vi "Virtualni instrument za merenje elektrofizioloskih signala.vi"() -> ()   [LabVIEW 2013]
uses:
  <vilib>/Instr/_visa.llb/VISA Configure Serial Port (Instr).vi
panel:
  out "Graficki prikaz rezultata":dbl(graph)
  in  "?":bool
  in  "Izbor porta":refnum<visa-resource-name>
  out "Broj rezultata":i32
  out "Lokacija sacuvanog fajla na racunaru":path
  in  "?":bool
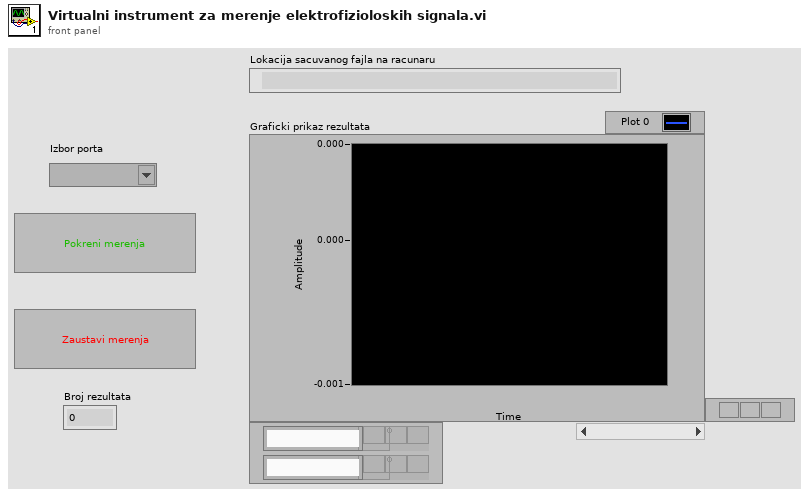
[diagram p1: front panel]
types:
  T1 = enum16{"open", "replace", "create", "open or create", "replace or create", "replace or create with confirmation"}
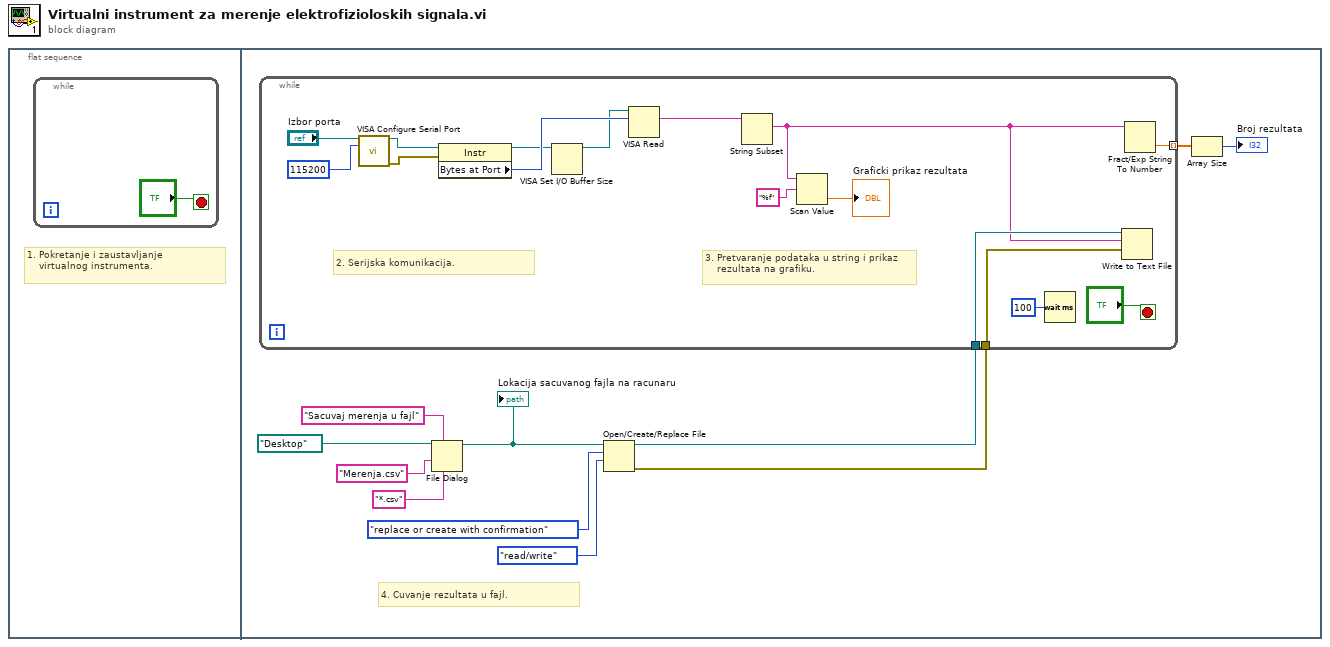
[diagram p0: block diagram]
diagram:
  n1 = flat-sequence {
    frame #0 {
      # "1. Pokretanje i zaustavljanje \n    virtualnog instrumenta."
      n2 = while {
        stop <- "?" stop-if-true
      }
    }
    frame #1 {
      # "4. Cuvanje rezultata u fajl."
      n3 = File Dialog(6:"*.csv" ("pattern (all files)"), 7:"Sacuvaj merenja u fajl" ("prompt"), 9:"Merenja.csv" ("default name"), 11:path "/Desktop" ("start path")) -> (3:w6:path)  [unwired: 1 in, 5 out]
      "Lokacija sacuvanog fajla na racunaru" <- w6
      n4 = Open/Create/Replace File(file path (use dialog)=w6, operation (0:open)=T1."replace or create with confirmation", access (0:read/write)=enum16{"read/write", "read-only", "write-only"}."read/write") -> (refnum out=w4:refnum<file>, error out=w3:errorcluster)  [unwired: 3 in, 1 out]
      n5 = while {
        tunnel: w4 -> [w26]
        tunnel: [w25] -> w2 mode=indexing
        tunnel: w3 -> [w24]
        stop <- "?" stop-if-true
        # "3. Pretvaranje podataka u string i prikaz\n    rezultata na grafiku."
        # "2. Serijska komunikacija."
        n6 = call-poly "VISA Configure Serial Port"("VISA resource name"="Izbor porta", "baud rate (9600)"=u32 115200) -> ("VISA resource name out"=w21:refnum<visa-resource-name>, "error out"=w20:errorcluster)  [unwired: 12 in]
        n7 = property class="Instr"(reference=w21, error in=w20) -> (reference out=w14:refnum<visa-resource-name>, "Bytes at Port"=w18:u32)  [unwired: 1 out]
        n8 = VISA Set I/O Buffer Size(VISA resource name=w14) -> (VISA resource name out=w13:refnum<visa-resource-name>)  [unwired: 3 in, 1 out]
        n9 = VISA Read(VISA resource name=w13, byte count=w18) -> (read buffer=w16:string)  [unwired: 1 in, 3 out]
        n10 = String Subset(string=w16) -> (substring=w22:string)  [unwired: 2 in]
        n11 = Scan Value(string=w22, format string="%f") -> (value=→"Graficki prikaz rezultata":dbl)  [unwired: 1 in, 1 out]
        n12 = Wait (ms)(milliseconds to wait=u32 100) -> ()  [unwired: 1 out]
        n13 = Write to Text File(file (use dialog)=w26, text=w22, error in=w24) -> ()  [unwired: 1 in, 3 out]
        n14 = Fract/Exp String To Number(string=w22) -> (number=w25:dbl)  [unwired: 3 in, 1 out]
      }
      n15 = Array Size(array=w2) -> (size(s)=→"Broj rezultata":i32)
    }
  }
